vi "UI_Control_System.vi"() -> ()   [LabVIEW 2014]
uses:
  Terminal-Global-SetValues.vi
panel:
  in  "停止":bool caption="启动"
  in  "系统执行状态":i32(listbox)
  out "右侧Y位移":dbl[](graph)
  out "右侧X位移":dbl[](graph)
  out "左侧Y位移":dbl[](graph)
  out "左侧X位移":dbl[](graph)
  out "齿轮子系统运行状态":bool
  out "动力子系统运行状态":bool
  out "DAQ采集运行状态":bool
  out "试验单元单元运行状态":bool
  out "陪试单元运行状态":bool
  out "加载单元运行状态":bool
  in  "加载单元查看详细":bool caption="加载单元"
  in  "主轴监测单元查看详细":bool caption="加载单元"
  in  "试验单元查看详细":bool caption="加载单元"
  in  "陪试单元查看详细":bool caption="加载单元"
  in  "实验进度":dbl(slide) scale=0.0..100.0 scale format="%#_g%%"
  out "Data":string caption="当前时间："
  out "系统当前状态":bool
  out "轴向位移幅度图":sgl[](graph)
  out "右侧轴心轨迹图":cluster{"电涡流3":sgl[], "电涡流4":sgl[]}(graph)
  out "左侧轴心轨迹图":cluster{"电涡流1":sgl[], "电涡流2":sgl[]}(graph)
  out "转速":sgl
  out "出油温度2":dbl
  out "出油温度1":dbl
  out "试验单元出油温度":dbl
  out "轴承外圈温度":dbl
  out "试验单元摩擦力矩":dbl
  out "声发射频谱图":sgl[](graph)
  out "声发射时间曲线":sgl[](graph)
  out "外壳振动频谱图":dbl(graph)
  out "外壳振动时间曲线":cluster{"加速度2":sgl[]}[](graph)
  out "轴向液压缸加载压力":dbl
  out "径向液压缸加载压力":dbl
  # "轴承测控系统"
  # "检测参数区域"
  # "主轴监测单元"
  # "加载单元"
  # "陪试单元"
  # "实验单元"
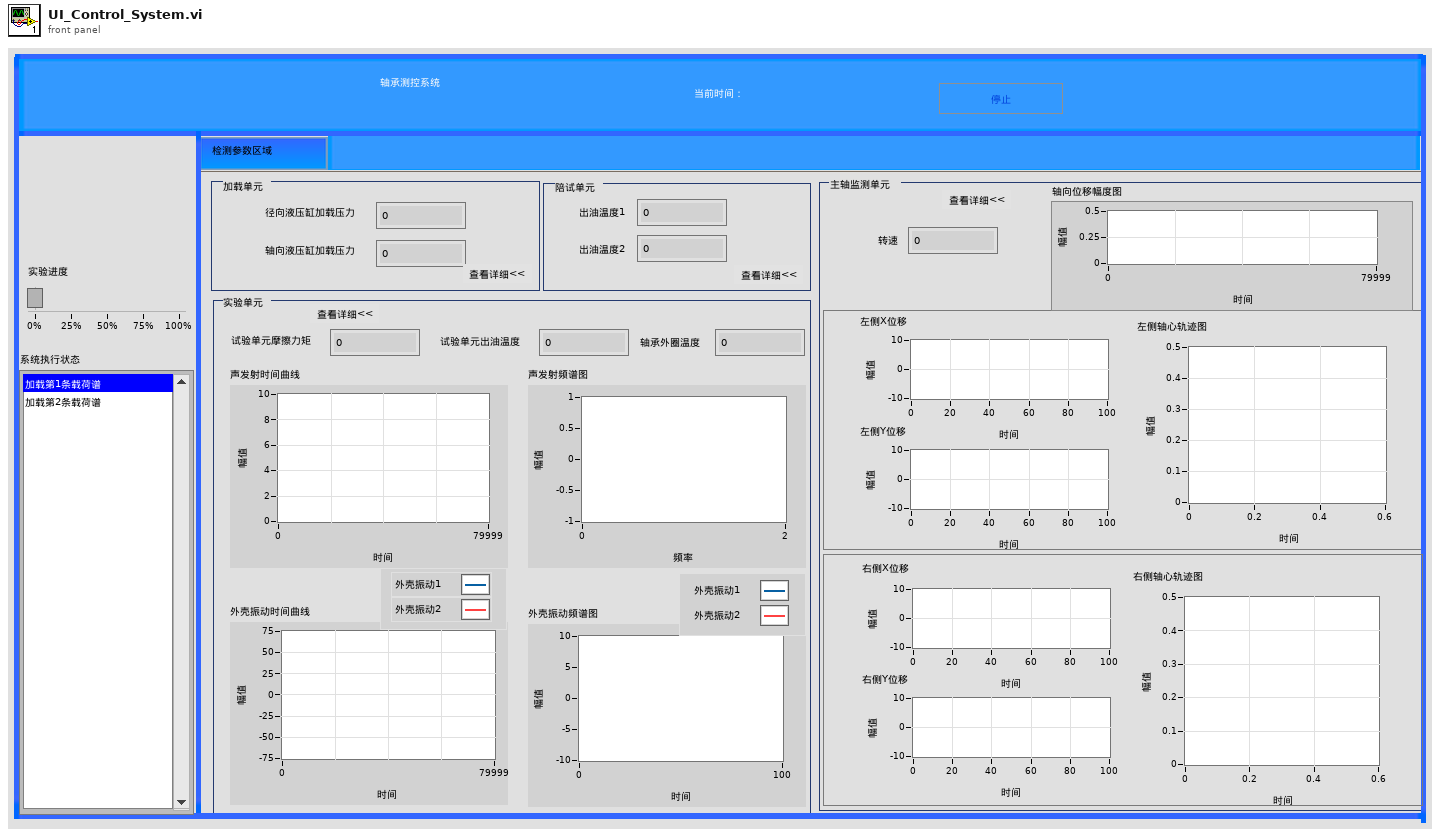
[diagram p1: front panel]
types:
  T1 = cluster{"时间":timestamp, "声发射":sgl[], "电涡流1":sgl[], "电涡流2":sgl[], "电涡流3":sgl[], "电涡流4":sgl[], "电涡流5":sgl[], "加速度1":sgl[], "加速度2":sgl[]}
  T2 = cluster{"时间":timestamp, "陪试轴承润滑单元出油温度1":sgl[], "陪试轴承润滑单元出油温度2":sgl[], "轴承外圈温度":sgl[], "出油温度":sgl[], "摩擦力1":sgl[], "摩擦力2":sgl[], "径向油缸力":sgl[], "轴向油缸力":sgl[], "转速":sgl[]}
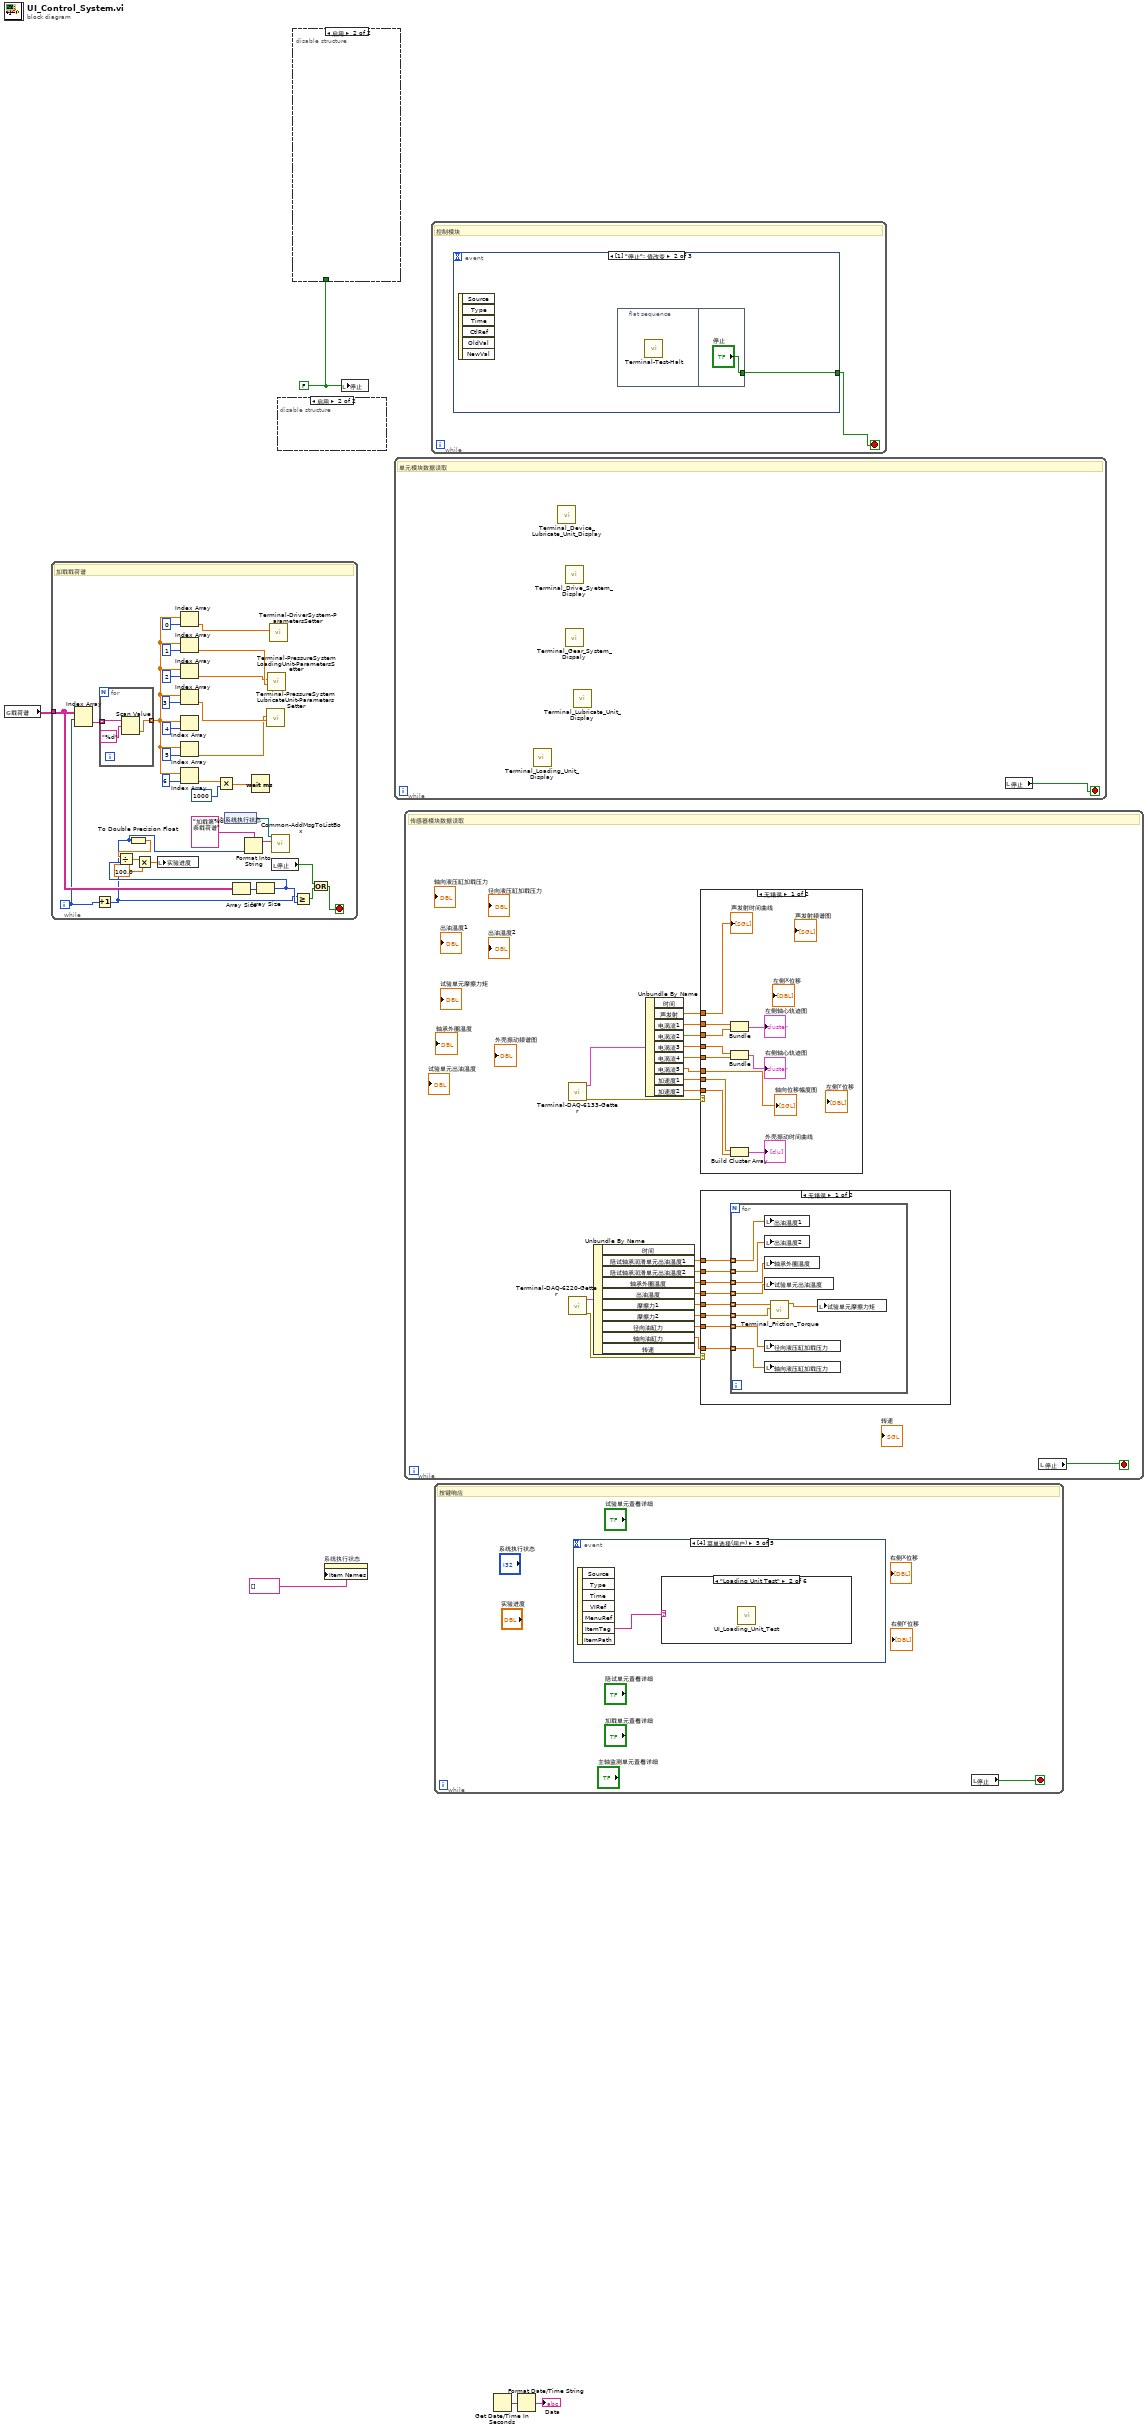
[diagram p0: block diagram]
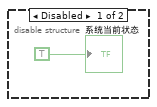
[diagram p2: hidden frame]
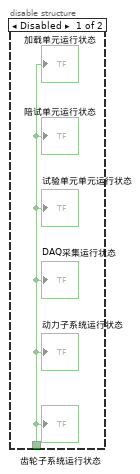
[diagram p3: hidden frame]
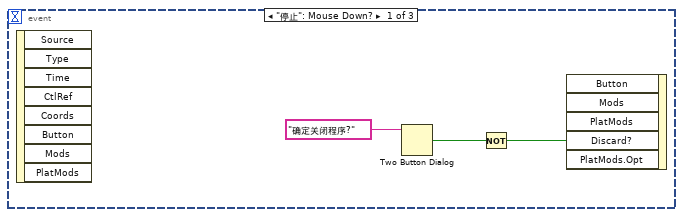
[diagram p6: hidden frame]
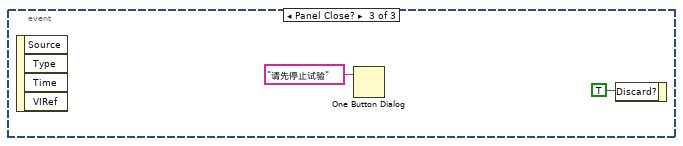
[diagram p7: hidden frame]
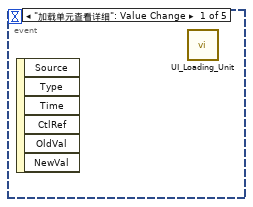
[diagram p8: hidden frame]
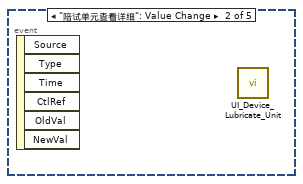
[diagram p9: hidden frame]
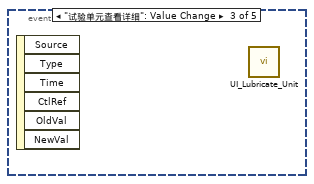
[diagram p10: hidden frame]
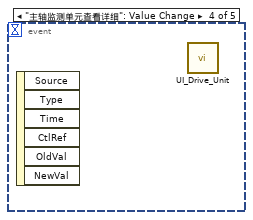
[diagram p11: hidden frame]
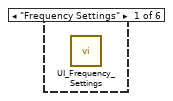
[diagram p12: hidden frame]
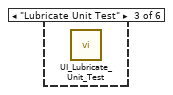
[diagram p13: hidden frame]
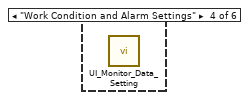
[diagram p14: hidden frame]
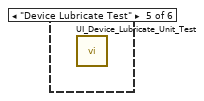
[diagram p15: hidden frame]
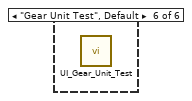
[diagram p16: hidden frame]
diagram:
  w3 = FALSE
  n1 = global read "Terminal-Global-SetValues.vi" "载荷谱"() -> (w2:string[][])
  n2 = while {
    tunnel: w2 -> [w18]
    i -> [w16]
    stop <- w11 stop-if-true
    # "加载载荷谱"
    n3 = Index Array(array=w18, index (row)=w16) -> (element=w37:string[])  [unwired: 1 in]
    n4 = Increment(x=w16) -> (x+1=w7:i32)
    n5 = for {
      tunnel: w37 -> [w40] mode=indexing
      tunnel: [w38] -> w36 mode=indexing
      n6 = Scan Value(string=w40, format string="%d" ("格式字符串")) -> (value=w38:dbl)  [unwired: 1 in, 1 out]
    }
    n7 = To Double Precision Float(number=w7) -> (double precision float=w14:dbl)
    n8 = Index Array(array=w36, index=0 ("索引")) -> (element=w23:dbl)
    n9 = Index Array(array=w36, index=1 ("索引")) -> (element=w22:dbl)
    n10 = Index Array(array=w36, index=2 ("索引")) -> (element=w21:dbl)
    n11 = Index Array(array=w36, index=3 ("索引")) -> (element=w20:dbl)
    n12 = Index Array(array=w36, index=4 ("索引")) -> ()  [unwired: 1 out]
    n13 = Index Array(array=w36, index=5 ("索引")) -> (element=w19:dbl)
    n14 = Index Array(array=w36, index=6 ("索引")) -> (element=w26:dbl)
    n15 = Multiply(x=w26, y=u32 1000 ("等待时间（毫秒）")) -> (x*y=w24:dbl)
    n16 = control-ref of="系统执行状态"() -> (w28:refnum<vi>)
    n17 = Array Size(array=w18) -> (size(s)=w17:i32[])
    n18 = Format Into String(format string="加载第%d条载荷谱" ("字符串"), w7) -> (resulting string=w27:string)  [unwired: 2 in, 1 out]
    n19 = Wait (ms)(milliseconds to wait=w24) -> ()  [unwired: 1 out]
    n20 = Array Size(array=w17) -> (size(s)=w15:i32)
    n21 = Divide(x=w14, y=w15) -> (x/y=w10:dbl)
    n22 = Multiply(x=w10, y=100.0) -> (x*y=w8:dbl)
    n23 = local write "实验进度"(w8) -> ()
    n24 = call "Terminal-PressureSystemLubricateUnit-ParametersSetter.vi"("供油润滑温度T"=w20, "供油流量L"=w19) -> ()  [unwired: 9 in, 1 out]
    n25 = call "Terminal-PressureSystemLoadingUnit-ParametersSetter.vi"("轴向载荷F2"=w22, "径向载荷F1"=w21) -> ()  [unwired: 9 in, 1 out]
    n26 = call "Terminal-DriverSystem-ParametersSetter.vi"("转速"=w23) -> ()  [unwired: 10 in, 1 out]
    n27 = call "Common-AddMsgToListBox.vi"("字符串"=w27, "列表框"=w28) -> ()  [unwired: 10 in]
    n28 = local read "停止"() -> (w6:bool)
    n29 = Greater Or Equal?(x=w7, y=w15) -> (x >= y?=w12:bool)
    n30 = Or(x=w6, y=w12) -> (x .or. y?=w11:bool)
  }
  n31 = disable-structure shown="启用" {
    frame Disabled {
      "系统当前状态" <- TRUE
    }
    frame Enabled {
    }
  }
  n32 = disable-structure shown="启用" {
    disable-tunnel: w3 -> [w42 _]
    frame Disabled {
      "加载单元运行状态" <- w42
      "陪试单元运行状态" <- w42
      "试验单元单元运行状态" <- w42
      "DAQ采集运行状态" <- w42
      "动力子系统运行状态" <- w42
      "齿轮子系统运行状态" <- w42
    }
    frame Enabled {
    }
  }
  n33 = property on="系统执行状态" class="LstBox (严格)"("Item Names"=string[] [] ("项名")) -> ()  [unwired: 2 in, 2 out]
  n34 = local write "停止"(w3) -> ()
  n35 = while {
    stop <- w43 stop-if-true
    # "单元模块数据读取"
    n36 = call "Terminal_Loading_Unit_Display.vi"() -> ()  [unwired: 12 in]
    n37 = call "Terminal_Device_Lubricate_Unit_Display.vi"() -> ()  [unwired: 12 in]
    n38 = call "Terminal_Drive_Syetem_Display.vi"() -> ()  [unwired: 12 in]
    n39 = call "Terminal_Gear_System_Dispaly.vi"() -> ()  [unwired: 12 in]
    n40 = call "Terminal_Lubricate_Unit_Display.vi"() -> ()  [unwired: 12 in]
    n41 = local read "停止"() -> (w43:bool)
  }
  n42 = while {
    stop <- w44 stop-if-true
    # "传感器模块数据读取"
    n43 = call "Terminal-DAQ-6133-Getter.vi"() -> ("error out"=w63:errorcluster, "6133"=w64:T1)  [unwired: 10 in]
    n44 = call "Terminal-DAQ-6220-Getter.vi"() -> ("error out"=w55:errorcluster, "6220"=w54:T2)  [unwired: 10 in]
    n45 = Unbundle By Name(w54) -> ("陪试轴承润滑单元出油温度1"=w52:sgl[], "陪试轴承润滑单元出油温度2"=w51:sgl[], "轴承外圈温度"=w50:sgl[], "出油温度"=w49:sgl[], "摩擦力1"=w48:sgl[], "摩擦力2"=w47:sgl[], "径向油缸力"=w53:sgl[], "轴向油缸力"=w46:sgl[])  [unwired: 2 out]
    n46 = Unbundle By Name(w64) -> ("声发射"=w60:sgl[], "电涡流1"=w62:sgl[], "电涡流2"=w61:sgl[], "电涡流3"=w59:sgl[], "电涡流4"=w58:sgl[], "电涡流5"=w45:sgl[], "加速度1"=w57:sgl[], "加速度2"=w56:sgl[])  [unwired: 1 out]
    n47 = case shown="无错误" w63 {
      tunnel: w60 -> [w83 _]
      tunnel: w62 -> [w92 _]
      tunnel: w61 -> [w91 _]
      tunnel: w57 -> [w87 _]
      tunnel: w56 -> [w84 _]
      tunnel: w59 -> [w88 _]
      tunnel: w58 -> [w85 _]
      tunnel: w45 -> [w82 _]
      frame No Error {
        n48 = Bundle("电涡流1"=w92, "电涡流2"=w91) -> (→"左侧轴心轨迹图":cluster{"电涡流1":sgl[], "电涡流2":sgl[]})  [unwired: 1 in]
        n49 = Bundle("电涡流3"=w88, "电涡流4"=w85) -> (→"右侧轴心轨迹图":cluster{"电涡流3":sgl[], "电涡流4":sgl[]})  [unwired: 1 in]
        n50 = Build Cluster Array(w87, w84) -> (→"外壳振动时间曲线":cluster{"加速度2":sgl[]}[])
        "轴向位移幅度图" <- w82
        "声发射时间曲线" <- w83
      }
      frame Error {
      }
    }
    n51 = case shown="无错误" w55 {
      tunnel: w53 -> [w72 _]
      tunnel: w52 -> [w71 _]
      tunnel: w51 -> [w70 _]
      tunnel: w50 -> [w69 _]
      tunnel: w49 -> [w68 _]
      tunnel: w48 -> [w67 _]
      tunnel: w47 -> [w66 _]
      tunnel: w46 -> [w65 _]
      frame No Error {
        n52 = for {
          tunnel: w72 -> [w81] mode=indexing
          tunnel: w71 -> [w80] mode=indexing
          tunnel: w70 -> [w79] mode=indexing
          tunnel: w69 -> [w78] mode=indexing
          tunnel: w68 -> [w77] mode=indexing
          tunnel: w67 -> [w76] mode=indexing
          tunnel: w66 -> [w75] mode=indexing
          tunnel: w65 -> [w73] mode=indexing
          n53 = local write "出油温度1"(w80) -> ()
          n54 = local write "出油温度2"(w79) -> ()
          n55 = local write "轴承外圈温度"(w78) -> ()
          n56 = local write "试验单元出油温度"(w77) -> ()
          n57 = local write "径向液压缸加载压力"(w81) -> ()
          n58 = local write "轴向液压缸加载压力"(w73) -> ()
          n59 = call "Terminal_Friction_Torque.vi"("摩擦力FR"=w75, "摩擦力FL"=w76) -> ("摩擦力矩"=w74:dbl)  [unwired: 9 in]
          n60 = local write "试验单元摩擦力矩"(w74) -> ()
        }
      }
      frame Error {
      }
    }
    n61 = local read "停止"() -> (w44:bool)
  }
  n62 = while {
    stop <- w93 stop-if-true
    # "控制模块"
    n63 = event shown="[1] \"停止\": 值改变" {
      selector: _ -> [_ _ _]
      dyn-events: _ -> [_ _ _]
      timeout: _ -> [_ _ _]
      tunnel: [_ w97 _] -> w93
      event "停止": Mouse Down? {
        n64 = event-data() -> ()  [unwired: 1 in, 8 out]
        n65 = Two Button Dialog(message="确定关闭程序?" ("消息")) -> (T button?=w95:bool)  [unwired: 2 in]
        n66 = Not(x=w95) -> (.not. x?=w94:bool)
        n67 = event-data("Discard?"=w94) -> ()  [unwired: 5 in, 1 out]
      }
      event "停止": Value Change {
        n68 = event-data() -> ()  [unwired: 1 in, 6 out]
        n69 = flat-sequence {
          tunnel: ["停止"] -> w97
          frame #0 {
            n70 = call "Terminal-Test-Halt.vi"() -> ()  [unwired: 11 in, 1 out]
          }
          frame #1 {
          }
        }
      }
      event Panel Close? {
        n71 = event-data() -> ()  [unwired: 1 in, 4 out]
        n72 = One Button Dialog(message="请先停止试验" ("消息")) -> ()  [unwired: 1 in, 1 out]
        n73 = event-data("Discard?"=TRUE ("放弃？")) -> ()  [unwired: 1 in, 1 out]
      }
    }
  }
  n74 = while {
    stop <- w101 stop-if-true
    # "按键响应"
    n75 = event shown="[4] 菜单选择(用户)" {
      selector: _ -> [_ _ _ _ _]
      dyn-events: _ -> [_ _ _ _ _]
      timeout: _ -> [_ _ _ _ _]
      event "加载单元查看详细": Value Change {
        n76 = event-data() -> ()  [unwired: 1 in, 6 out]
        n77 = call "UI_Loading_Unit.vi"() -> ()  [unwired: 12 in]
      }
      event "陪试单元查看详细": Value Change {
        n78 = event-data() -> ()  [unwired: 1 in, 6 out]
        n79 = call "UI_Device_Lubricate_Unit.vi"() -> ()  [unwired: 12 in]
      }
      event "试验单元查看详细": Value Change {
        n80 = event-data() -> ()  [unwired: 1 in, 6 out]
        n81 = call "UI_Lubricate_Unit.vi"() -> ()  [unwired: 12 in]
      }
      event "主轴监测单元查看详细": Value Change {
        n82 = event-data() -> ()  [unwired: 1 in, 6 out]
        n83 = call "UI_Drive_Unit.vi"() -> ()  [unwired: 12 in]
      }
      event Menu Selection (User) {
        n84 = event-data() -> ("ItemTag"=w102:string)  [unwired: 1 in, 6 out]
        n85 = case shown="\"Loading Unit Test\"" w102 {
          frame "Frequency Settings" {
            n86 = call "UI_Frequency_Settings.vi"() -> ()  [unwired: 12 in]
          }
          frame "Loading Unit Test" {
            n87 = call "UI_Loading_Unit_Test.vi"() -> ()  [unwired: 12 in]
          }
          frame "Lubricate Unit Test" {
            n88 = call "UI_Lubricate_Unit_Test.vi"() -> ()  [unwired: 12 in]
          }
          frame "Work Condition and Alarm Settings" {
            n89 = call "UI_Monitor_Data_Setting.vi"() -> ()  [unwired: 12 in]
          }
          frame "Device Lubricate Test" {
            n90 = call "UI_Device_Lubricate_Unit_Test.vi"() -> ()  [unwired: 12 in]
          }
          frame "Gear Unit Test", Default {
            n91 = call "UI_Gear_Unit_Test.vi"() -> ()  [unwired: 12 in]
          }
        }
      }
    }
    n92 = local read "停止"() -> (w101:bool)
  }
  n93 = Get Date/Time In Seconds() -> (seconds since 1Jan1904=w4:timestamp)
  n94 = Format Date/Time String(seconds (now)=w4) -> (date/time string=→"Data":string)  [unwired: 2 in]
